vi "fake tool no description.vi"() -> ()   [LabVIEW 2020, in "MCP Server tests.lvlib"]
uses:
  MCP Server tests.lvlib
panel:
  out "string out":string
  in  "string in":string
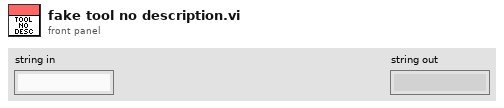
[diagram p1: front panel]
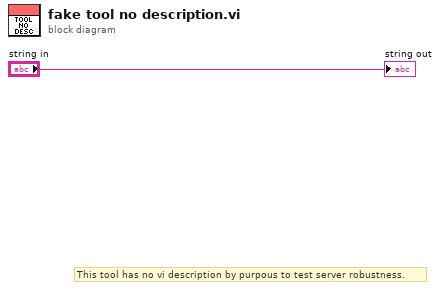
[diagram p0: block diagram]
diagram:
  # "This tool has no vi description by purpous to test server robustness."
  "string out" <- "string in"
